vi "gwyscan save gwyddion arrays.vi"(0 "data IN":dbl[](array[numeric]), 1 "nchannels":i32, 2 "xres":i32, 3 "yres":i32, 4 "xreal":dbl, 5 "yreal":dbl, 7 "error in (no error)":errorcluster, 8 "filename":string, 9 "xyunit":u64[](array[numeric]), 11 "zunit":u64[](array[numeric]), 13 "description":u64[](array[numeric])) -> (20 "data out":dbl[](array[numeric]), 21 "function return":i32, 22 "filename out":string, 27 "error out":errorcluster)   [LabVIEW 2016, in "libgwyscan.lvlib"]
doc: "GWYSCANDLL_API int gwyscan_save_gwyddion_arrays(double *data, int nchannels, int xres, int yres, double xreal, double yreal, char **xyunit, char **zunit, char **description, char *filename);"
uses:
  libgwyscan.lvlib
  libgwyscan.dll
panel:
  in  "Tab Control":enum32{"Main", "Error"}(tab)
  out "xyunit 2":i32[](array[numeric])
  out "zunit 2":i32[](array[numeric])
  out "description 2":i32[](array[numeric])
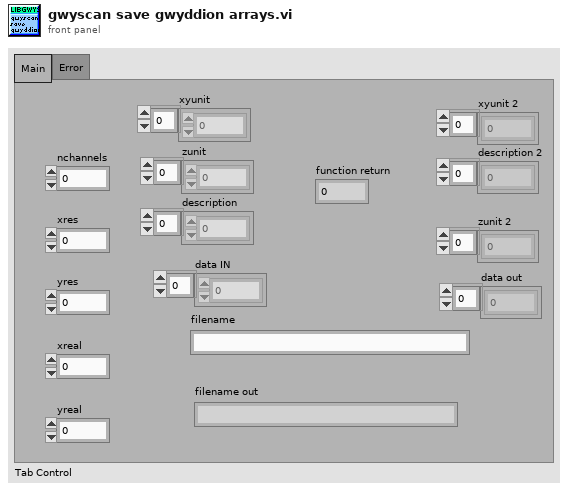
[diagram p1: front panel]
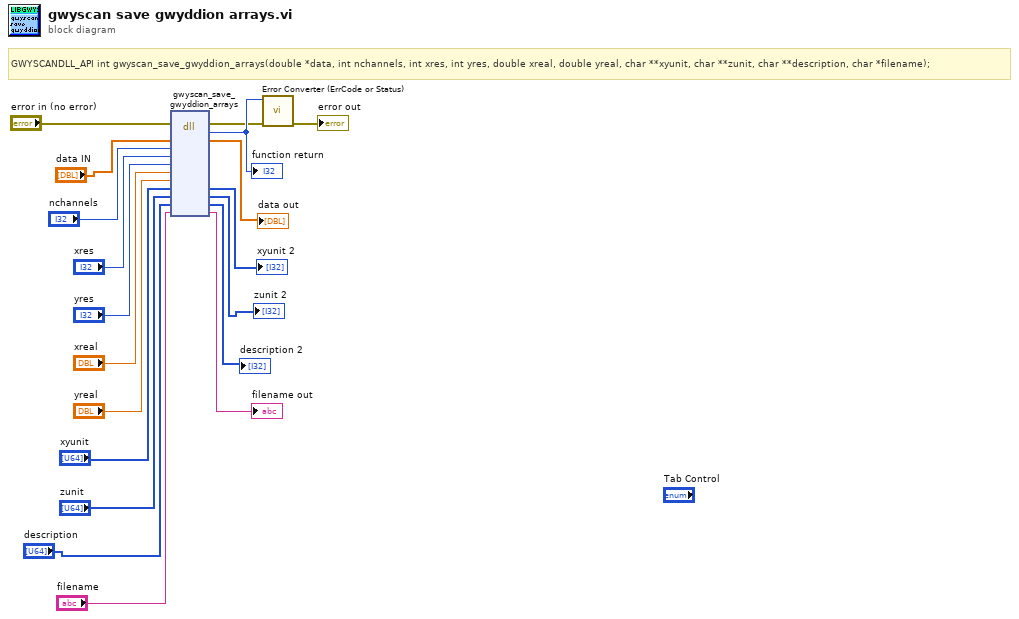
[diagram p0: block diagram]
diagram:
  # "GWYSCANDLL_API int gwyscan_save_gwyddion_arrays(double *data, int nchannels, int xres, int yres, double xreal, double yreal, char **xyunit, char **zunit, char **description, char *filename);"
  n1 = dll-call lib="PTH2’abs CUsersCharlÃ¨ne BrillardDesktoplbni-lbniAFMController-BetaVersionv2.0.16-20190611 libgwyscan-1.2-labview2015-win32libgwyscan.dll" fn="gwyscan_save_gwyddion_arrays"(error in="error in (no error)", "data"="data IN", "nchannels"="nchannels", "xres"="xres", "yres"="yres", "xreal"="xreal", "yreal"="yreal", "xyunit"="xyunit", "zunit"="zunit", "description"="description", "filename"="filename") -> (error out=w7:errorcluster, "return type"=w19:i32, "data"=→"data out":dbl[], "xyunit"=→"xyunit 2":i32[], "zunit"=→"zunit 2":i32[], "description"=→"description 2":i32[], "filename"=→"filename out":string)  [unwired: 7 in, 1 out]
  "function return" <- w19
  n2 = call "Error Converter (ErrCode or Status).vi"("error in (no error)"=w7, "error code"=w19) -> ("error out"=→"error out":errorcluster)  [unwired: 9 in]
